vi "Basic Messaging.vi"() -> (3 "Pass?":bool)   [LabVIEW 2014]
uses:
  TestActor/TestActor.lvclass
  <vilib>/ActorFramework/LastAck/Last Ack.lvclass
  <vilib>/ActorFramework/Message Queue/Message Queue.lvclass/Message Queue.ctl
  Increment Msg/Increment Msg.lvclass/Increment Msg.ctl
  <vilib>/ActorFramework/Message Enqueuer/Message Enqueuer.lvclass/Message Enqueuer.ctl
  <vilib>/ActorFramework/Message Dequeuer/Message Dequeuer.lvclass/Message Dequeuer.ctl
  <vilib>/ActorFramework/LastAck/Last Ack.lvclass/Last Ack.ctl
  TestActor/TestActor.lvclass/TestActor.ctl
  <vilib>/ActorFramework/Message Enqueuer/Enqueue.vi
  <vilib>/ActorFramework/Message Priority Queue/Priority Dequeue.vi
  <vilib>/ActorFramework/Message Priority Queue/Priority Enqueue.vi
  Increment Msg/Increment Msg.lvclass
  <vilib>/ActorFramework/Stop Msg/Stop Msg.lvclass
  <vilib>/ActorFramework/Actor/Actor.lvclass
  <vilib>/ActorFramework/Message Queue/Message Queue.lvclass
  <vilib>/ActorFramework/Message Dequeuer/Message Dequeuer.lvclass
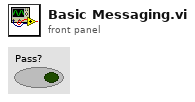
[diagram p1: front panel]
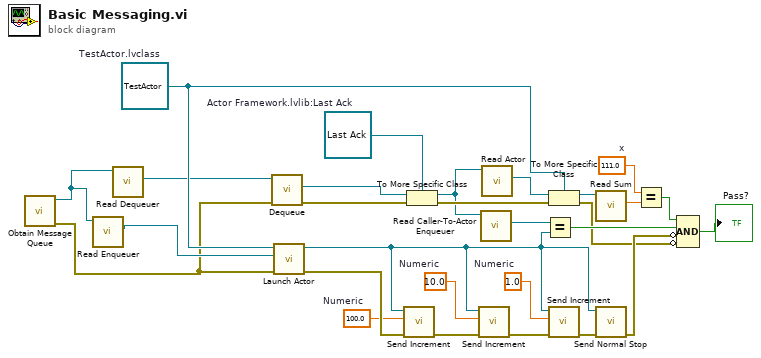
[diagram p0: block diagram]
diagram:
  w14 = 111.0  # x
  w21 = refnum<class "Last Ack.lvclass"> refnum  # Actor Framework.lvlib:Last Ack
  w23 = 1.0  # Numeric
  w25 = 10.0  # Numeric
  w27 = 100.0  # Numeric
  w17 = refnum<class "TestActor.lvclass"> refnum  # TestActor.lvclass
  n1 = call <vilib>:"Obtain Message Queue.vi"() -> ("error out"=w4:errorcluster, "Message Queue"=w7:refnum<class "Message Queue.lvclass">)  [unwired: 10 in]
  n2 = call <vilib>:"Read Enqueuer.vi"("Message Queue"=w7) -> ("Message Enqueuer"=w8:refnum<class "Message Enqueuer.lvclass">)  [unwired: 10 in]
  n3 = call <vilib>:"Read Dequeuer.vi"("Message Queue"=w7) -> ("Message Dequeuer"=w6:refnum<class "Message Dequeuer.lvclass">)  [unwired: 10 in]
  n4 = call <vilib>:"Dequeue.vi"("error in (no error)"=w4, "Message Dequeuer in"=w6) -> ("error out"=w3:errorcluster, "Message"=w5:refnum<class "Message.lvclass">)  [unwired: 5 in, 3 out]
  n5 = call <vilib>:"Launch Actor.vi"("error in (no error)"=w4, "Actor-to-Caller Enqueuer"=w8, "Actor"=w17) -> ("error out"=w28:errorcluster, "Caller-To-Actor Enqueuer"=w20:refnum<class "Message Enqueuer.lvclass">)  [unwired: 7 in]
  n6 = call "Send Increment.vi"("error in (no error)"=w28, "Numeric"=w27, "Actor Framework.lvlib:Send Queue"=w20) -> ("error out"=w26:errorcluster)  [unwired: 8 in]
  n7 = To More Specific Class(target class=w21, reference=w5, error in=w3) -> (specific class reference=w1:refnum<class "Last Ack.lvclass">, error out=w19:errorcluster)
  n8 = call "Send Increment.vi"("error in (no error)"=w26, "Numeric"=w25, "Actor Framework.lvlib:Send Queue"=w20) -> ("error out"=w24:errorcluster)  [unwired: 8 in]
  n9 = call <vilib>:"Read Caller-To-Actor Enqueuer.vi"("Last Ack"=w1) -> ("Caller-to-Actor Enqueuer"=w2:refnum<class "Message Enqueuer.lvclass">)  [unwired: 10 in]
  n10 = call <vilib>:"Read Actor.vi"("Last Ack"=w1) -> ("Actor"=w18:refnum<class "Actor.lvclass">)  [unwired: 10 in]
  n11 = Equal?(x=w2, y=w20) -> (x = y?=w12:bool)
  n12 = To More Specific Class(target class=w17, reference=w18, error in=w19) -> (specific class reference=w16:refnum<class "TestActor.lvclass">, error out=w9:errorcluster)
  n13 = call "Send Increment.vi"("error in (no error)"=w24, "Numeric"=w23, "Actor Framework.lvlib:Send Queue"=w20) -> ("error out"=w22:errorcluster)  [unwired: 8 in]
  n14 = call "Read Sum.vi"("TestActor in"=w16) -> ("Sum"=w15:dbl)  [unwired: 9 in, 1 out]
  n15 = call <vilib>:"Send Normal Stop.vi"("error in (no error)"=w22, "Message Enqueuer"=w20) -> ("error out"=w10:errorcluster)  [unwired: 9 in]
  n16 = Equal?(x=w14, y=w15) -> (x = y?=w13:bool)
  n17 = Compound Arithmetic op=AND(w13, w12, invert w10, invert w9) -> (→"Pass?":bool)
